vi "Memory.Pointer.Clear Subset.Unsafe.vi"(8 "error in (no error)":errorcluster, 9 "offset (0)":u64 format="%08x bytes", 10 "length":u64 format="%08x bytes", 11 "pointer in":refnum<class "Memory.Pointer.lvclass">) -> (0 "error out":errorcluster, 3 "pointer out":refnum<class "Memory.Pointer.lvclass">)   [LabVIEW 2016, in "Memory Manager.lvlib" / "Memory.Pointer.lvclass"]
doc: "Sets the subset of bytes specified by <b>offset</b> and <b>length</b> within the provided <b>pointer</b> to zero.\n\n<b>Note:</b> This VI is <b>unsafe</b>, meaning it does not performs null pointer and bounds checks to prevent invaid memory access. Invalid arguments provided to this method can crash or corrupt LabVIEW memory."
uses:
  Memory.Pointer.lvclass
  Memory.Pointer.lvclass/Memory.Pointer.ctl
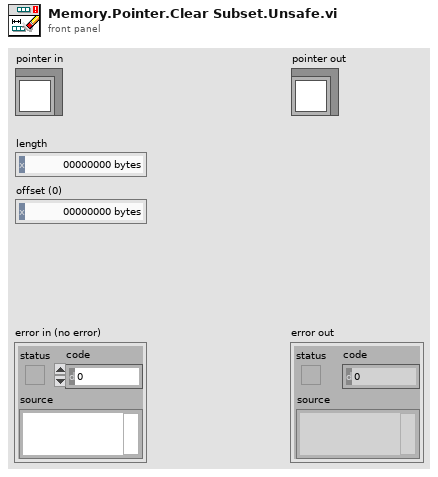
[diagram p1: front panel]
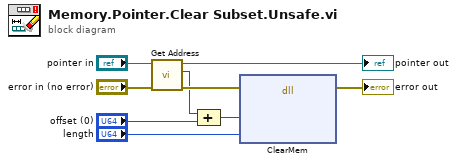
[diagram p0: block diagram]
diagram:
  n1 = call "Get Address.vi"("error in (no error)"="error in (no error)", "Pointer in"="pointer in") -> ("error out"=w9:errorcluster, "address"=w6:u64, "Pointer out"=→"pointer out":refnum<class "Memory.Pointer.lvclass">)  [unwired: 7 in]
  n2 = Compound Arithmetic op=ADD(w6, "offset (0)") -> (w5:u64)
  n3 = dll-call lib="LabVIEW" fn="ClearMem"(error in=w9, "pointer"=w5, "size"="length") -> (error out=→"error out":errorcluster)  [unwired: 5 in, 1 out]
